vi "button_event_test.vi"() -> ()   [LabVIEW 2020]
uses:
  Subs/Server XCtrl/Server.xctl
  Subs/Console XCtrl/Console_Xctrl.xctl
panel:
  out "REPL":string(xcontrol)
  in  "Clear":bool
  in  "Server":bool
  in  "Help":bool
  in  "Server":path(xcontrol)=path "/Users/crogers/GitHub/Summer2020/LabVIEWCode/Servers/Jens.vi"
  in  "Move motor":bool
  in  "stop":bool
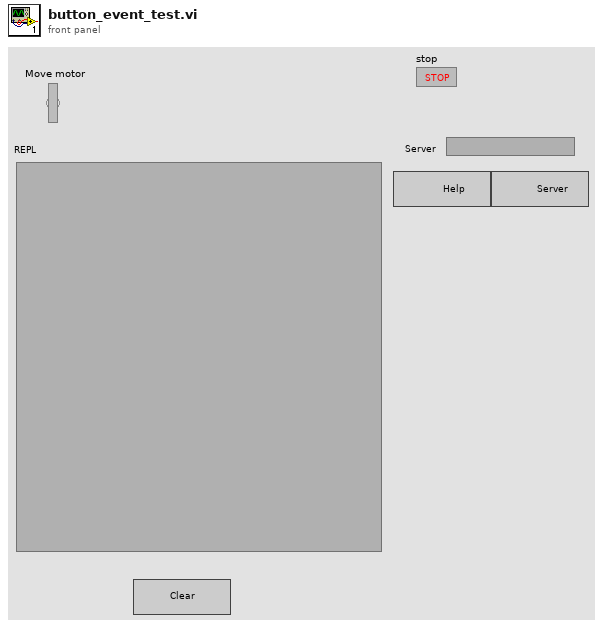
[diagram p1: front panel]
types:
  T1 = enum8{"Enabled", "Disabled", "Disabled and Grayed Out"}
  T2 = typedef "eventvkey.ctl" = enum16{"ASCII", "Enter", "Return", "Shift", "Ctrl", "Alt", "Cmd", "Opt", "Caps", "NumLock", "Clear", "Break", "Up", "Down", "Left", "Right", "Insert", "Delete", "Home", "End", "PageUp", "PageDown", "Escape", "Help", "Pause", "ScrollLock", "F1", "F2", "F3", "F4", "F5", "F6", "F7", "F8", "F9", "F10", "F11", "F12", "F13", "F14", "F15", "F16", "F17", "F18", "F19", "F20", "F21", "F22", "F23", "F24", "Play", "VolumeUp", "VolumeDown", "Mute", "Two Byte Char"}
  T3 = cluster{"Shift":bool, "Ctrl":bool, "Alt":bool, "Cmd":bool, "Opt":bool}
  T4 = cluster{"Char":i16, "VKey":T2, "PlatMods":cluster{"Shift":bool, "Ctrl":bool, "Alt":bool, "Cmd":bool, "Opt":bool}}
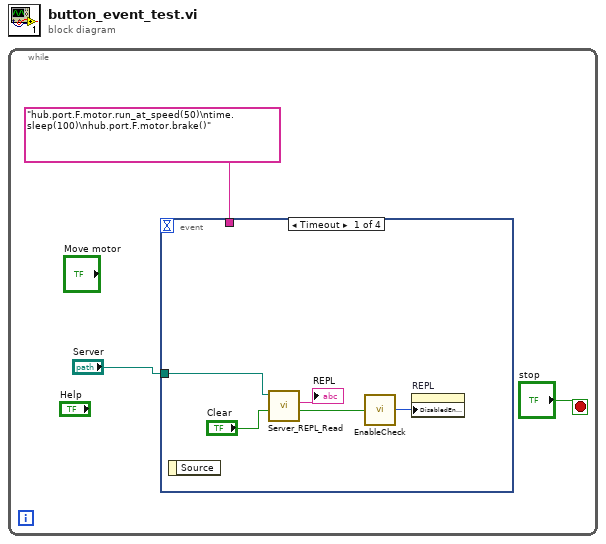
[diagram p0: block diagram]
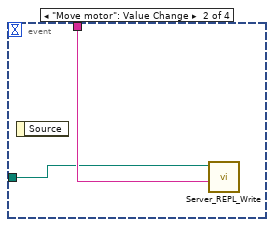
[diagram p2: hidden frame]
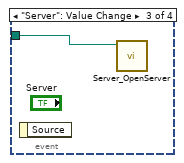
[diagram p3: hidden frame]
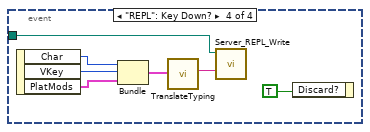
[diagram p4: hidden frame]
diagram:
  n1 = while {
    stop <- "stop" stop-if-true
    n2 = event shown="[0] Timeout" {
      selector: _ -> [_ _ _ _]
      dyn-events: _ -> [_ _ _ _]
      timeout: _ -> [_ _ _ _]
      tunnel: "Server" -> [w4 w9 w11 w12]
      tunnel: "hub.port.F.motor.run_at_speed(50)\ntime.sleep(100)\nhub.port.F.motor.brake()" -> [_ w10 _ _]
      event Timeout {
        n3 = event-data() -> ()  [unwired: 1 in, 1 out]
        n4 = call "Server_REPL_Read.vi"("Clear"="Clear", "Server"=w4) -> ("Running?"=w7:bool, "REPL"=→"REPL":string)  [unwired: 7 in, 1 out]
        n5 = call "EnableCheck.vi"("Enable?"=w7) -> ("Enum"=w8:T1)
        n6 = property on="REPL" class="Console_Xctrl (strict)"("DisabledEnum"=w8) -> ()  [unwired: 2 in, 2 out]
      }
      event "Move motor": Value Change {
        n7 = event-data() -> ()  [unwired: 1 in, 1 out]
        n8 = call "Server_REPL_Write.vi"("Code"=w10, "Server"=w9) -> ()  [unwired: 9 in, 1 out]
      }
      event "Server": Value Change {
        n9 = event-data() -> ()  [unwired: 1 in, 1 out]
        n10 = call "Server_OpenServer.vi"("Server"=w11) -> ()  [unwired: 10 in, 1 out]
      }
      event "REPL": Key Down? {
        n11 = event-data() -> ("Char"=w15:i16, "VKey"=w14:T2, "PlatMods"=w13:T3)  [unwired: 1 in]
        n12 = Bundle("Char"=w15, "VKey"=w14, "PlatMods"=w13) -> (w18:T4)  [unwired: 1 in]
        n13 = call "TranslateTyping.vi"("Cluster"=w18) -> ("key"=w17:string)  [unwired: 10 in]
        n14 = call "Server_REPL_Write.vi"("Code"=w17, "Server"=w12) -> ()  [unwired: 9 in, 1 out]
        n15 = event-data("Discard?"=TRUE) -> ()  [unwired: 1 in, 1 out]
      }
    }
  }
